vi "NewData.vi"(6 "Instance":i32, 8 "error in (no error)":errorcluster, 11 "Data":dbl[][](array[numeric])) -> (0 "error out":errorcluster)   [LabVIEW 2017, in "Chart.lvlib"]
uses:
  Chart.lvlib
  NewData.Data.ctl
  Communication/Communication.lvlib
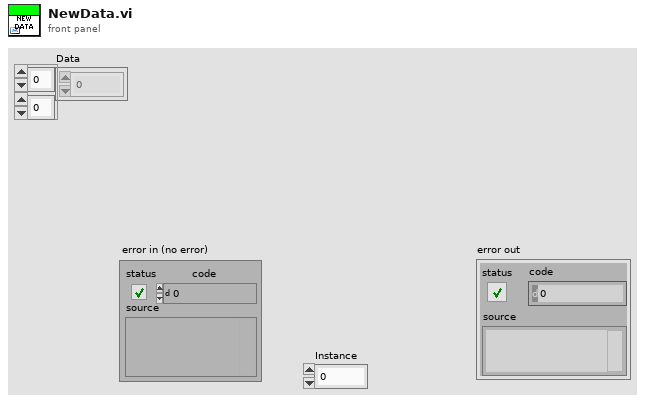
[diagram p1: front panel]
types:
  T1 = typedef "Chart.lvlib/NewData.Data.ctl" = cluster{"Data":dbl[][]}
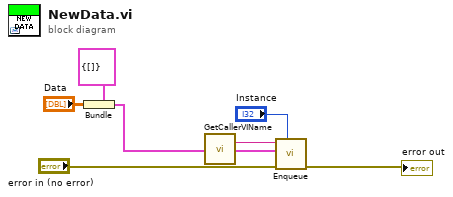
[diagram p0: block diagram]
diagram:
  n1 = Bundle(cluster=T1 {"Data"=[]}, "Data"="Data") -> (w4:T1)
  n2 = call "GetCallerVIName.vi"() -> ("VI name"=w2:string)  [unwired: 11 in]
  n3 = call "Enqueue.vi"("Instance"="Instance", "error in (no error)"="error in (no error)", "Data"=w4, "Msg"=w2) -> ("error out"=→"error out":errorcluster)  [unwired: 7 in]
